vi "XZ to angle and hyoptenuse.vi"(6 "Arm Offset (Inches)":dbl, 8 "Z":dbl, 11 "X":dbl) -> (0 "Hypotenuse (Inches)":dbl, 3 "Angle (degrees)":dbl)   [LabVIEW 2023]
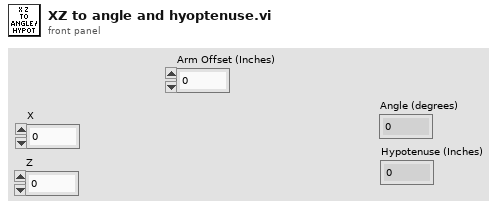
[diagram p1: front panel]
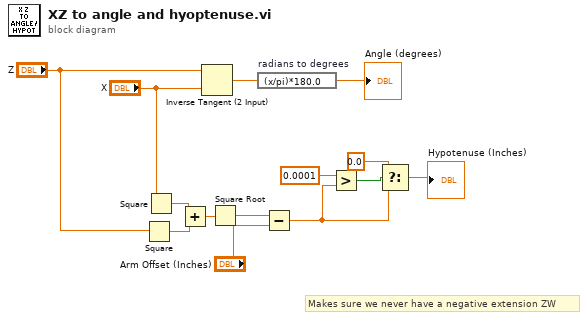
[diagram p0: block diagram]
diagram:
  # "Makes sure we never have a negative extension ZW"
  n1 = Square(x="Z") -> (x^2=w13:dbl)
  n2 = Square(x="X") -> (x^2=w14:dbl)
  n3 = Add(x=w14, y=w13) -> (x+y=w12:dbl)
  n4 = Inverse Tangent (2 Input)(1:"X", 2:"Z") -> (0:w9:dbl)
  n5 = Square Root(x=w12) -> (sqrt(x)=w7:dbl)
  n6 = expression code="(x/pi)*180.0" "radians to degrees"(w9) -> (→"Angle (degrees)":dbl)
  n7 = Subtract(x=w7, y="Arm Offset (Inches)") -> (x-y=w2:dbl)
  n8 = Greater?(x=0.0001, y=w2) -> (0:w4:bool)
  n9 = Select(t=0.0, s=w4, f=w2) -> (s? t:f=→"Hypotenuse (Inches)":dbl)
